vi "Tetra_ADC-Frame.vi"(0 "COMPORT":refnum<visa-resource-name>="COM4", 11 "error in (no error)":errorcluster, 12 "Execute":bool, 13 "Open Ser(t)":bool, 14 "Close Ser(t)":bool) -> (2 "locked(t)":bool, 3 "chan_id":string, 4 "comport":refnum<visa-resource-name>="COM4", 15 "error out":errorcluster)   [LabVIEW 2018]
panel:
  out "chan_id":dbl[](array[numeric])
  out "Success":bool
  out "output":string="\r"
  in  "Command":string="adcframe"
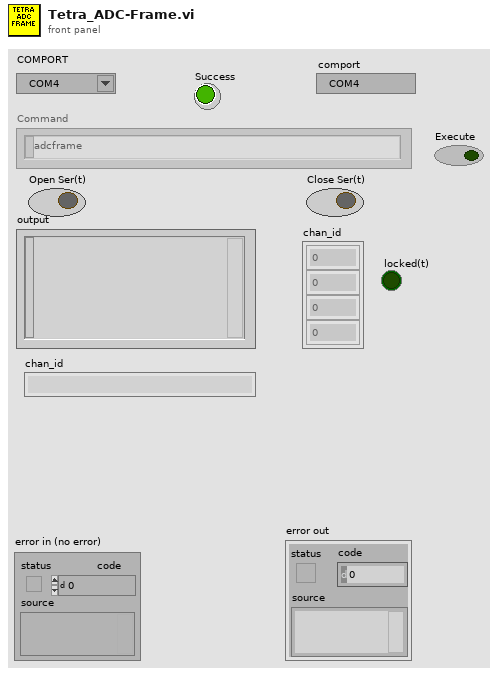
[diagram p1: front panel]
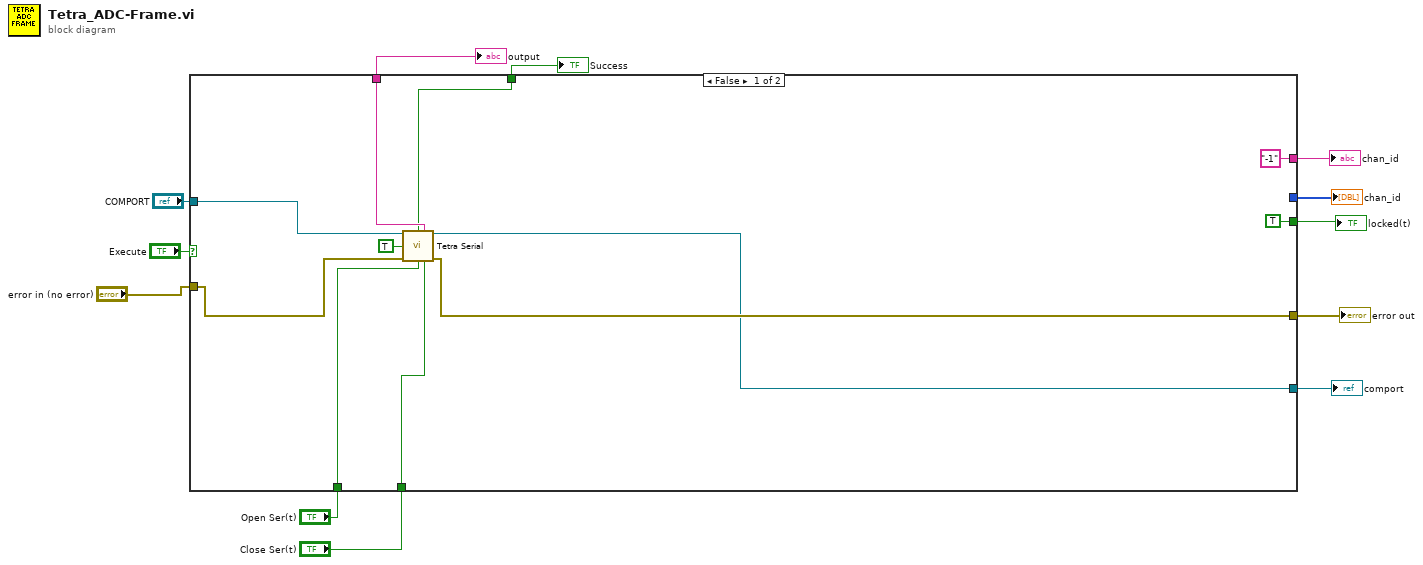
[diagram p0: block diagram]
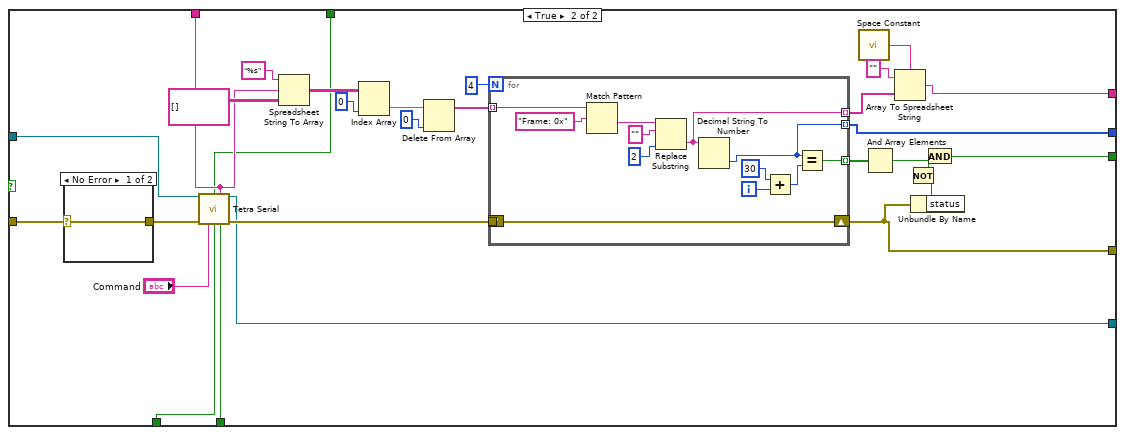
[diagram p2: hidden frame]
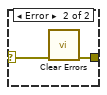
[diagram p3: hidden frame]
diagram:
  n1 = case shown="False" "Execute" {
    tunnel: "error in (no error)" -> [w21 w38]
    tunnel: [w20 w35] -> w11
    tunnel: "Close Ser(t)" -> [w15 w32]
    tunnel: "Open Ser(t)" -> [w16 w31]
    tunnel: "COMPORT" -> [w18 w30]
    tunnel: [w19 w29] -> w6
    tunnel: [_ w28] -> w5
    tunnel: ["-1" ("spreadsheet string") w27] -> w4
    tunnel: [w23 w26] -> w3
    tunnel: [w22 w25] -> w2
    tunnel: [TRUE w24] -> w1
    frame False {
      n2 = call "Tetra Serial.vi"("COMPORT"=w18, "ClearErrorIn(t)"=TRUE, "error in (no error)"=w21, "Open Ser(t)"=w16, "Close Ser(t)"=w15) -> ("Success"=w22:bool, "output"=w23:string, "comport"=w19:refnum<visa-resource-name>, "error out"=w20:errorcluster)  [unwired: 6 in, 1 out]
    }
    frame True {
      n3 = case shown="No Error" w38 {
        selector: w38 -> [w53 w55]
        tunnel: [w53 w54] -> w37
        frame No Error {
        }
        frame Error {
          n4 = call <vilib>:"Clear Errors.vi"("error in (no error)"=w55) -> ("error out"=w54:errorcluster)  [unwired: 5 in, 1 out]
        }
      }
      n5 = call "Tetra Serial.vi"("COMPORT"=w30, "error in (no error)"=w37, "Command"="Command", "Open Ser(t)"=w31, "Close Ser(t)"=w32) -> ("Success"=w25:bool, "output"=w26:string, "comport"=w29:refnum<visa-resource-name>, "error out"=w36:errorcluster)  [unwired: 6 in, 1 out]
      n6 = Spreadsheet String To Array(format string="%s", spreadsheet string=w26, array type (2D Dbl)=string[][] []) -> (array=w49:string[][])  [unwired: 1 in]
      n7 = Index Array(array=w49, index (col)=0 ("disabled index (col)")) -> (element=w47:string[])  [unwired: 1 in]
      n8 = Delete From Array(array=w47, index=0) -> (array with subset deleted=w46:string[])  [unwired: 1 in, 1 out]
      n9 = for {
        N: 4 -> [_]
        tunnel: w46 -> [w67] mode=indexing
        tunnel: [w60] -> w28 mode=indexing
        tunnel: [w58] -> w43 mode=indexing
        tunnel: [w57] -> w42 mode=indexing
        tunnel: w36 -> [w56]
        shift-right: [w56] -> w35
        shift-left: _ -> [_]
        i -> [w61]
        n10 = Match Pattern(string=w67, regular expression="Frame: 0x") -> (after substring=w65:string)  [unwired: 1 in, 3 out]
        n11 = Replace Substring(2:2 ("length (len. of substring)"), 4:"" ("substring (\"\")"), 5:w65) -> (0:w57:string)  [unwired: 1 in, 1 out]
        n12 = Decimal String To Number(string=w57) -> (number=w60:i32)  [unwired: 2 in, 1 out]
        n13 = Add(x=30, y=w61) -> (x+y=w62:i32)
        n14 = Equal?(x=w60, y=w62) -> (x = y?=w58:bool)
      }
      n15 = call <vilib>:"Space Constant.vi"() -> ("String"=w41:string)
      n16 = And Array Elements(Boolean array=w43) -> (logical AND=w39:bool)
      n17 = Array To Spreadsheet String(delimiter (Tab)=w41, array=w42, 3:"" ("format string")) -> (spreadsheet string=w27:string)
      n18 = Unbundle By Name(w35) -> ("status"=w34:bool)
      n19 = Not(x=w34) -> (.not. x?=w33:bool)
      n20 = And(x=w33, y=w39) -> (x .and. y?=w24:bool)
    }
  }
  "error out" <- w11
  "comport" <- w6
  "chan_id" <- w5
  "chan_id" <- w4
  "output" <- w3
  "Success" <- w2
  "locked(t)" <- w1
